vi "Read formula_info.vi"(8 "error in (no error)":errorcluster, 11 "Alicat_P in":refnum<class "P.lvclass">) -> (0 "error out":errorcluster, 2 "formula_info":cluster{"Table":i32[][], "Y Values":dbl[]} {"Y Values" format="%.2f"}, 3 "Alicat_P out":refnum<class "P.lvclass">)   [LabVIEW 2013, in "Alicat.lvlib" / "P.lvclass"]
uses:
  P.lvclass
  P.lvclass/P.ctl
panel:
  # "operator"
  # "register1"
  # "register2"
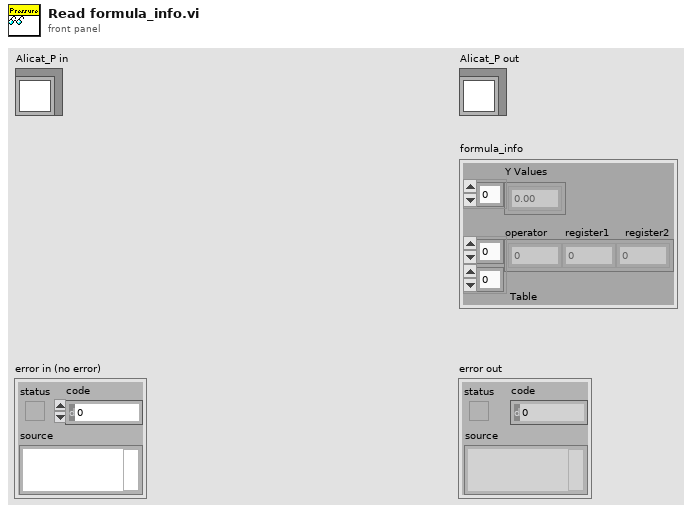
[diagram p1: front panel]
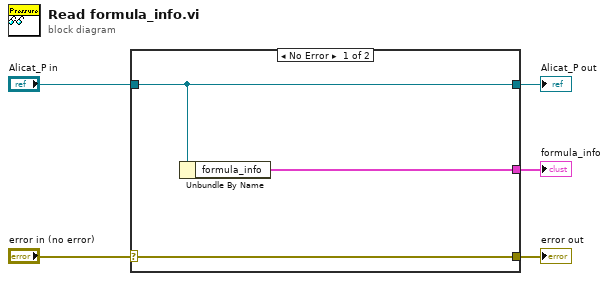
[diagram p0: block diagram]
diagram:
  n1 = case shown="No Error" "error in (no error)" {
    selector: "error in (no error)" -> [w8 w9]
    tunnel: [w8 w9] -> w4
    tunnel: [w7 w10] -> w2
    tunnel: "Alicat_P in" -> [w7 w10]
    tunnel: [w6 _] -> w1
    frame No Error {
      n2 = Unbundle By Name(w7) -> ("formula_info"=w6:cluster{"Table":i32[][], "Y Values":dbl[]})
    }
    frame Error {
    }
  }
  "error out" <- w4
  "Alicat_P out" <- w2
  "formula_info" <- w1
